vi "Test_No Error.vi"(8 "error in (no error)":errorcluster, 11 "TestCase in":refnum<class "Construct.lvclass">=refnum) -> (0 "error out":errorcluster, 3 "TestCase out":refnum<class "Construct.lvclass">)   [LabVIEW 2017, in "Construct.lvclass"]
uses:
  Construct.lvclass
  Source/User Configuration Manager Ref/By Ref.lvlib
  Source/User Configuration Manager/User Configuration Manager.lvclass
  C:/Users/huijun.guo/Desktop/composed-user-manager/Source/iUser Configuration Manager/iUser Configuration Manager.lvclass
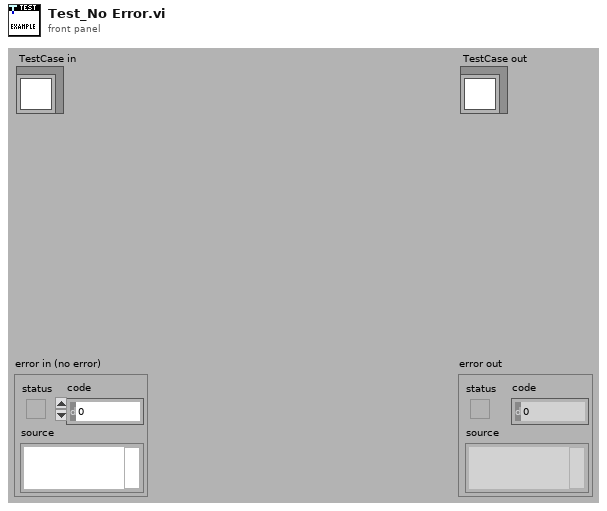
[diagram p1: front panel]
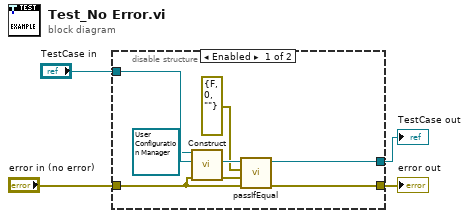
[diagram p0: block diagram]
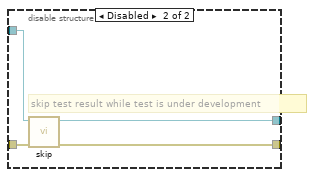
[diagram p2: hidden frame]
diagram:
  n1 = disable-structure "This diagram is for convenience to enable skipping a test easily (enable 'Skip' case)" shown="Enabled" {
    disable-tunnel: "TestCase in" -> [w11 w15]
    disable-tunnel: [w10 w13] -> w1
    disable-tunnel: [w9 w14] -> w3
    disable-tunnel: "error in (no error)" -> [w6 w12]
    frame Enabled {
      n2 = call "Construct.vi"("iUser Configuration Manager in"=refnum<class "User Configuration Manager.lvclass"> refnum ("User Configuration Manager.lvlib:User Configuration Manager"), "error in"=w6) -> ("error out"=w7:errorcluster)  [unwired: 12 in, 1 out]
      n3 = call-dynamic "passIfEqual.vi"("error in (no error)"=w6, "y"=w7, "x"=errorcluster {"status"=FALSE, "code"=0, "source"=""} ("error out"), "TestCase in"=w11) -> ("error out"=w9:errorcluster, "TestCase out"=w10:refnum<class "Construct.lvclass">)  [unwired: 6 in]
    }
    frame Disabled {
      # "skip test result while test is under development"
      n4 = call <vilib>:"skip.vi"("error in (no error)"=w12, "TestCase in"=w15) -> ("error out"=w14:errorcluster, "TestCase out"=w13:refnum<class "Construct.lvclass">)  [unwired: 8 in]
    }
  }
  "error out" <- w3
  "TestCase out" <- w1
